vi "Read Multi Numeric as CDBL.vi"(8 "error in (no error)":errorcluster, 9 "Type":cdb[](array[numeric]), 10 "Tag":string[](array[string]), 11 "Var Bus in":refnum<class "Omni_Bus.lvclass">) -> (0 "error out":errorcluster, 2 "Array":cdb[](array[numeric]), 3 "Var Bus out":refnum<class "Omni_Bus.lvclass">)   [LabVIEW 2021, in "Omni_Bus.lvclass"]
uses:
  Omni_Bus.lvclass
  <vilib>/TSA/Abstract Data Classes/Abs_Types/Numeric/Abs_Numeric.lvclass
  Omni_Bus.lvclass/Omni_Bus.ctl
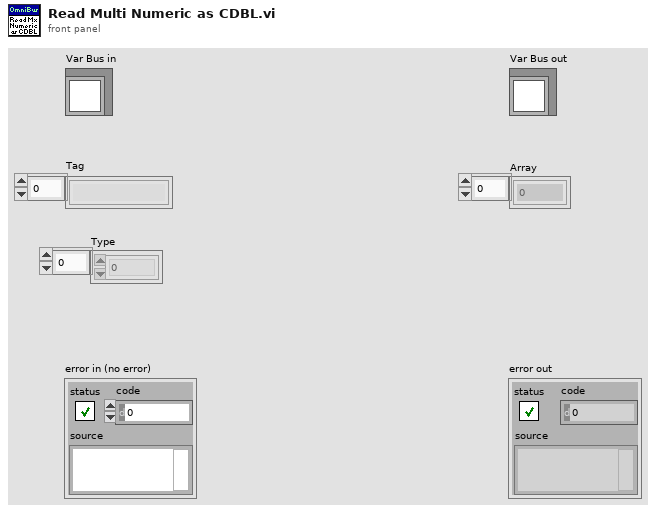
[diagram p1: front panel]
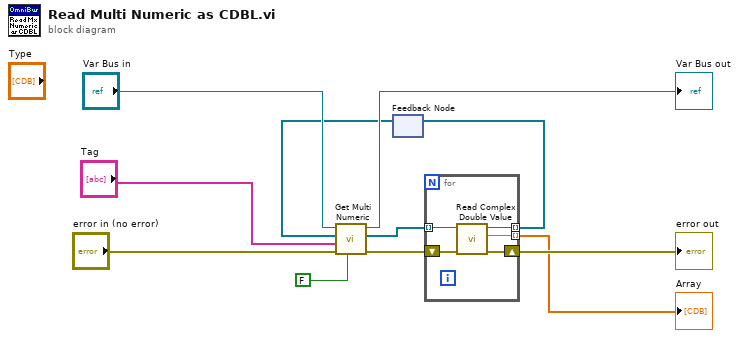
[diagram p0: block diagram]
diagram:
  n1 = feedback #1() -> (w2:refnum<class "Abs_Numeric.lvclass">[])  [unwired: 1 in]
  n2 = call-dynamic "Get Multi Numeric.vi"("Write?"=FALSE, "error in (no error)"="error in (no error)", "Tag"="Tag", "Value Type"=w2, "Var Bus in"="Var Bus in") -> ("error out"=w4:errorcluster, "Value Out"=w3:refnum<class "Abs_Numeric.lvclass">[], "Var Bus out"=→"Var Bus out":refnum<class "Omni_Bus.lvclass">)  [unwired: 4 in]
  n3 = for {
    tunnel: [w15] -> w6 mode=indexing
    tunnel: [w14] -> w5 mode=indexing
    tunnel: w3 -> [w12] mode=indexing
    shift-right: [w16] -> w10
    shift-left: w4 -> [w13]
    n4 = call-dynamic "Read Complex Double Value.vi"("error in (no error)"=w13, "Numeric in"=w12) -> ("error out"=w16:errorcluster, "Complex Double Float"=w15:cdb, "Numeric out"=w14:refnum<class "Abs_Numeric.lvclass">)  [unwired: 7 in]
  }
  "error out" <- w10
  "Array" <- w6
  n5 = feedback-in #1(w5) -> ()
